vi "ADO Recordset Open.vi"(0 "ADODB._Recordset In":refnum<k7>, 1 "ADODB._Connection In":refnum<k7>, 2 "CursorType":i32(ring)=-1 items=["adOpenUnspecified"=-1, "adOpenForwardOnly"=0, "adOpenKeyset"=1, "adOpenDynamic"=2, "adOpenStatic"=3], 3 "LockType":i32(ring)=-1 items=["adLockUnspecified"=-1, "adLockReadOnly"=1, "adLockPessimistic"=2, "adLockOptimistic"=3, "adLockBatchOptimistic"=4], 4 "Options":i32, 5 "error in (no error)":errorcluster, 7 "Command Text":string) -> (14 "ADODB._Recordset Out":refnum<k7>, 19 "error out":errorcluster)   [LabVIEW 2013]
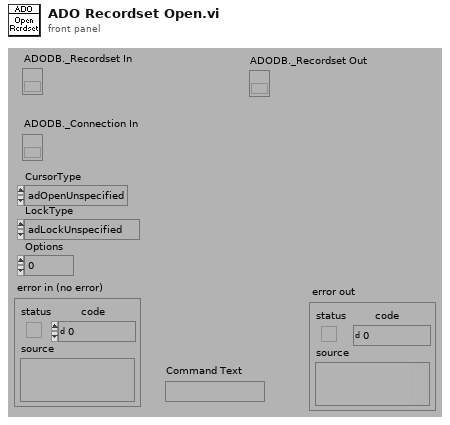
[diagram p1: front panel]
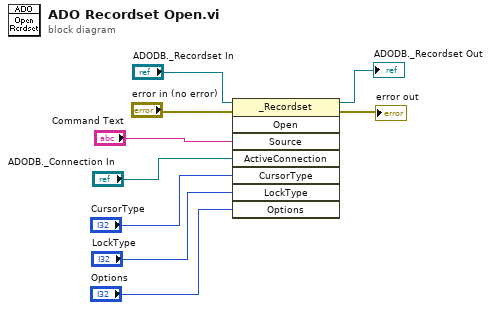
[diagram p0: block diagram]
diagram:
  n1 = invoke class="_Recordset" method="Open"(reference="ADODB._Recordset In", error in="error in (no error)", "Source"="Command Text", "ActiveConnection"="ADODB._Connection In", "CursorType"="CursorType", "LockType"="LockType", "Options"="Options") -> (reference out=→"ADODB._Recordset Out":refnum<k7>, error out=→"error out":errorcluster)  [unwired: 1 in, 6 out]
